vi "Find Speeds and Angles.vi"(5 "Prev Angles":dbl[](array[numeric]), 6 "Gyro Angle":dbl, 7 "Twist Axis":dbl, 8 "Y Axis":dbl, 9 "X Axis":dbl) -> (0 "Speeds":dbl[](array[numeric]), 3 "Angles":dbl[](array[numeric]))   [LabVIEW 2020]
doc: "Performs all calculations necessary for the implementation of Swerve Drive.\n\n X Axis:\nThe X Axis of Driving Joystick (Strafing). Range: [-1, 1].\n Y Axis:\nThe X Axis of Driving Joystick (Strafing). Range: [-1, 1].\n Twist Axis:\nThe Twist Axis of Driving Joystick (Twist). Range: [-1, 1].\n Gyro:\nAngle of Gyro 0. Range: [0, 360].\n Previous Angles:\nList of angles of each wheel as measured by the absolute encode. Ranges [0, 360]"
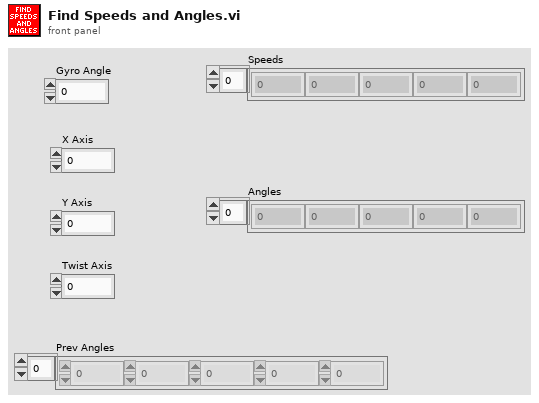
[diagram p1: front panel]
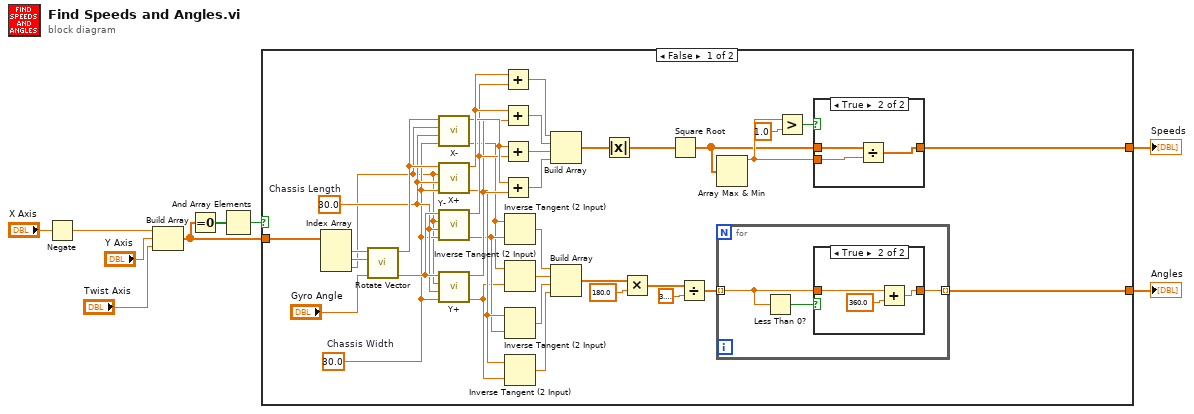
[diagram p0: block diagram]
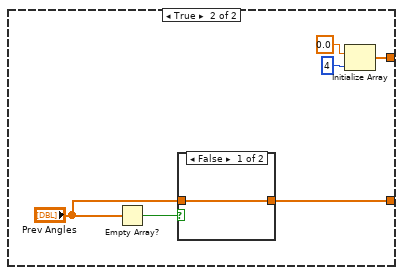
[diagram p4: hidden frame]
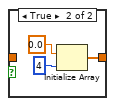
[diagram p5: hidden frame]
diagram:
  n1 = Negate(x="X Axis") -> (-x=w1:dbl)
  n2 = Build Array(w1, "Y Axis", "Twist Axis") -> (w8:dbl[])
  n3 = Equal To 0?(x=w8) -> (x = 0?=w7:bool[])
  n4 = And Array Elements(Boolean array=w7) -> (logical AND=w6:bool)
  n5 = case shown="False" w6 {
    tunnel: w8 -> [w16 _]
    tunnel: [w12 w59] -> w5
    tunnel: [w11 w63] -> w4
    frame False {
      w21 = 30.0  # Chassis Width
      w22 = 30.0  # Chassis Length
      n6 = Index Array(array=w16) -> (element #1=w15:dbl, element #2=w14:dbl, element #3=w13:dbl)  [unwired: 3 in]
      n7 = call "Rotate Vector.vi"("Angle"="Gyro Angle", "Y"=w14, "X"=w15) -> ("Y'"=w23:dbl, "X'"=w24:dbl)  [unwired: 7 in]
      n8 = call "X-.vi"("Width"=w21, "Length"=w22, "Z"=w13, "X"=w24) -> ("X-"=w40:dbl, "(X-)^2"=w45:dbl)  [unwired: 6 in]
      n9 = call "X+.vi"("Width"=w21, "Length"=w22, "Z"=w13, "X"=w24) -> ("X+"=w42:dbl, "(X+)^2"=w46:dbl)  [unwired: 6 in]
      n10 = call "Y-.vi"("Width"=w21, "Length"=w22, "Z"=w13, "Y"=w23) -> ("Y-"=w41:dbl, "(Y-)^2"=w44:dbl)  [unwired: 6 in]
      n11 = call "Y+.vi"("Width"=w21, "Length"=w22, "Z"=w13, "Y"=w23) -> ("Y+"=w39:dbl, "(Y+)^2"=w43:dbl)  [unwired: 6 in]
      n12 = Add(x=w46, y=w44) -> (x+y=w20:dbl)
      n13 = Add(x=w46, y=w43) -> (x+y=w19:dbl)
      n14 = Add(x=w45, y=w44) -> (x+y=w18:dbl)
      n15 = Add(x=w45, y=w43) -> (x+y=w17:dbl)
      n16 = Inverse Tangent (2 Input)(1:w41, 2:w40) -> (0:w35:dbl)
      n17 = Inverse Tangent (2 Input)(1:w39, 2:w40) -> (0:w34:dbl)
      n18 = Inverse Tangent (2 Input)(1:w41, 2:w42) -> (0:w33:dbl)
      n19 = Inverse Tangent (2 Input)(1:w39, 2:w42) -> (0:w32:dbl)
      n20 = Build Array(w20, w19, w18, w17) -> (w38:dbl[])
      n21 = Build Array(w35, w34, w33, w32) -> (w31:dbl[])
      n22 = Absolute Value(x=w38) -> (abs(x)=w26:dbl[])
      n23 = Multiply(x=w31, y=180.0) -> (x*y=w29:dbl[])
      n24 = Square Root(x=w26) -> (sqrt(x)=w25:dbl[])
      n25 = Divide(x=w29, y=3.141592653589793) -> (x/y=w27:dbl[])
      n26 = Array Max & Min(array=w25) -> (max value=w37:dbl)  [unwired: 3 out]
      n27 = for {
        tunnel: w27 -> [w49] mode=indexing
        tunnel: [w48] -> w11 mode=indexing
        n28 = Less Than 0?(x=w49) -> (x < 0?=w50:bool)
        n29 = case shown="True" w50 {
          tunnel: w49 -> [w51 w54]
          tunnel: [w51 w52] -> w48
          frame False {
          }
          frame True {
            n30 = Add(x=w54, y=360.0) -> (x+y=w52:dbl)
          }
        }
      }
      n31 = Greater?(x=w37, y=1.0) -> (0:w36:bool)
      n32 = case shown="True" w36 {
        tunnel: w25 -> [w55 w58]
        tunnel: w37 -> [_ w56]
        tunnel: [w55 w57] -> w12
        frame False {
        }
        frame True {
          n33 = Divide(x=w58, y=w56) -> (x/y=w57:dbl[])
        }
      }
    }
    frame True {
      n34 = Empty Array?(array="Prev Angles") -> (empty?=w64:bool)
      n35 = case shown="False" w64 {
        tunnel: [w65 w68] -> w63
        tunnel: "Prev Angles" -> [w65 _]
        frame False {
        }
        frame True {
          n36 = Initialize Array(0.0 ("element"), 4 ("dimension size")) -> (w68:dbl[])
        }
      }
      n37 = Initialize Array(0.0 ("element"), 4 ("dimension size")) -> (w59:dbl[])
    }
  }
  "Speeds" <- w5
  "Angles" <- w4
